vi "Read Integral.vi"(0 "VISA resource name":refnum<visa-resource-name>, 1 "Data Source (0: Data Trace)":u16(ring) items=["Data Trace", "Memory Trace"], 11 "error in (no error)":errorcluster, 12 "Maximum Time (10000 ms)":u32=10000) -> (2 "Integrated Noise (dBc)":dbl format="%^#_9g", 3 "Frequency Range (Hz)":dbl format="%^#_9g", 4 "VISA resource name out":refnum<visa-resource-name>, 6 "RMS Noise (deg)":dbl format="%^#_9g", 8 "RMS Jitter (s)":dbl format="%^#_9g", 10 "Residual FM (Hz)":dbl format="%^#_9g", 14 "RMS Noise (rad)":dbl format="%^#_9g", 15 "error out":errorcluster)   [LabVIEW 2011, in "Agilent E5052X.lvlib"]
doc: "Reads the integrated phase noise, frequency range, RMS noise, RMS jitter, and residual FM Frequency Modulation of data and memory trace data. \n\n<b>Note: </b>\n\nThis VI only applies to Phase Noise measurements."
uses:
  Agilent E5052X.lvlib
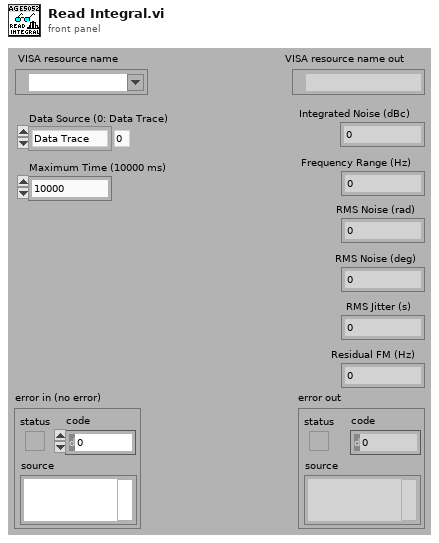
[diagram p1: front panel]
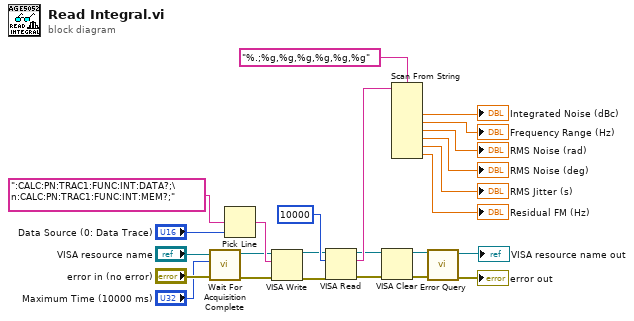
[diagram p0: block diagram]
diagram:
  n1 = call "Wait For Acquisition Complete.vi"("error in (no error)"="error in (no error)", "Maximum Time (10000)"="Maximum Time (10000 ms)", "VISA resource name"="VISA resource name") -> ("error out"=w6:errorcluster, "VISA resource name out"=w7:refnum<visa-resource-name>)  [unwired: 7 in]
  n2 = Pick Line(multi-line string=":CALC:PN:TRAC1:FUNC:INT:DATA?;\n:CALC:PN:TRAC1:FUNC:INT:MEM?;", line index="Data Source (0: Data Trace)") -> (output string=w11:string)  [unwired: 1 in]
  n3 = VISA Write(VISA resource name=w7, write buffer=w11, error in (no error)=w6) -> (VISA resource name out=w13:refnum<visa-resource-name>, error out=w12:errorcluster)  [unwired: 1 out]
  n4 = VISA Read(VISA resource name=w13, byte count=u32 10000, error in (no error)=w12) -> (VISA resource name out=w16:refnum<visa-resource-name>, read buffer=w24:string, error out=w15:errorcluster)  [unwired: 1 out]
  n5 = VISA Clear(VISA resource name=w16, error in (no error)=w15) -> (VISA resource name out=w2:refnum<visa-resource-name>, error out=w1:errorcluster)
  n6 = Scan From String(format string="%.;%g,%g,%g,%g,%g,%g", input string=w24) -> (output 1=→"Integrated Noise (dBc)":dbl, output 2=→"Frequency Range (Hz)":dbl, output 3=→"RMS Noise (rad)":dbl, output 4=→"RMS Noise (deg)":dbl, output 5=→"RMS Jitter (s)":dbl, output 6=→"Residual FM (Hz)":dbl)  [unwired: 8 in, 3 out]
  n7 = call "Error Query.vi"("error in (no error)"=w1, "VISA resource name"=w2) -> ("error out"=→"error out":errorcluster, "VISA resource name out"=→"VISA resource name out":refnum<visa-resource-name>)  [unwired: 6 in, 2 out]
